vi "svfa_Compute Zoom FFT.vi"(0 "x":dbl[](array[numeric]) format="%.2f", 1 "processing control":T9(ring), 2 "spectrum info":T1={"channel name"="", "description"="", "x-axis units"=0, "spectral info"={"spectrum type"=enum."Power [Magnitude^2]", "linear/dB"=enum."linear", "window"=0, "window size"=0, "FFT size"=0}, "engineering units"=0, "custom label"="", "dB reference [EU]"=0.0, "peak units"=enum."rms", "weighting filter"=0, "spectral density?"=FALSE, "unit label"="", "spectrum skewed?"=FALSE, "complimentary spectrum units"=enum."none"} {"x-axis units" items=["Time (s)"=0, "Frequency-CB (Hz)"=1, "Frequency-CPB (Hz)"=1248, "Frequency-Arbitrary (Hz)"=2357, "Quefrency (s)"=2, "Revolutions (rev)"=3, "Order"=4, "Speed (RPM)"=11, "Speed (rad/s)"=21, "Index"=65535]; "weighting filter" items=["Linear", "A-weighting", "B-weighting", "C-weighting", "ITU-R 468-4", "Dolby", "CCITT", "C-message", "Wb", "Wc", "Wd", "We", "Wf", "Wh", "Wj", "Wk", "Wm", "AES17 20 kHz lowpass", "AES17 40 kHz lowpass", "AES17 20 kHz highpass", "AES17 40 kHz highpass"]; "dB reference [EU]" format="%.2f"; "engineering units" items=["custom..."=0, "V"=1, "A"=21, "C"=30, "pC"=31, "s"=32, "-"=29, "Pa"=2, "N"=20, "g"=3, "m/s^2"=4, "m/s"=5, "m"=6, "mm/s"=12, "mm"=13, "micron/s"=14, "micron"=15, "in/s^2"=7, "in/s"=8, "in"=9, "mil/s"=10, "mil"=11, "rad/s^2"=16, "rad/s"=17, "rad"=18, "deg/s^2"=26, "deg/s"=27, "deg"=28, "RPM"=22, "cycle/s^2"=23, "Hz"=24, "cycle"=25, "strain"=19]; "spectral info"."window" items=["None "=0, "Hanning"=1, "Hamming"=2, "Blackman-Harris"=3, "Exact Blackman"=4, "Blackman"=5, "Flat Top"=6, "4 Term B-Harris "=7, "7 Term B-Harris"=8, "Low Sidelobe"=9, "Force - Exponential"=10, "Gaussian"=62]}, 5 "fs":dbl=1024.0 format="%.2f", 9 "zoom FFT settings":T8={"zoom settings"={"center frequency"=-inf, "zoom"=1, "trim"=1.0}, "FFT settings"={"window"=enum."Hanning", "window size"=-1, "FFT size"=1024, "%overlap"=0.0}} {"FFT settings"."%overlap" min=0.0 max=100.0 format="%.2f"; "zoom settings"."trim" min=1.0 format="%.2f"; "zoom settings"."center frequency" format="%.2f"; "zoom settings"."zoom" min=1}, 11 "error in (no error)":errorcluster, 13 "export time data?":bool) -> (3 "spectrum info out":T1={"channel name"="", "description"="", "x-axis units"=0, "spectral info"={"spectrum type"=enum."Power [Magnitude^2]", "linear/dB"=enum."linear", "window"=0, "window size"=0, "FFT size"=0}, "engineering units"=0, "custom label"="", "dB reference [EU]"=0.0, "peak units"=enum."rms", "weighting filter"=0, "spectral density?"=FALSE, "unit label"="", "spectrum skewed?"=FALSE, "complimentary spectrum units"=enum."none"} {"x-axis units" items=["Time (s)"=0, "Frequency-CB (Hz)"=1, "Frequency-CPB (Hz)"=1248, "Frequency-Arbitrary (Hz)"=2357, "Quefrency (s)"=2, "Revolutions (rev)"=3, "Order"=4, "Speed (RPM)"=11, "Speed (rad/s)"=21, "Index"=65535]; "weighting filter" items=["Linear", "A-weighting", "B-weighting", "C-weighting", "ITU-R 468-4", "Dolby", "CCITT", "C-message", "Wb", "Wc", "Wd", "We", "Wf", "Wh", "Wj", "Wk", "Wm", "AES17 20 kHz lowpass", "AES17 40 kHz lowpass", "AES17 20 kHz highpass", "AES17 40 kHz highpass"]; "dB reference [EU]" format="%.2f"; "engineering units" items=["custom..."=0, "V"=1, "A"=21, "C"=30, "pC"=31, "s"=32, "-"=29, "Pa"=2, "N"=20, "g"=3, "m/s^2"=4, "m/s"=5, "m"=6, "mm/s"=12, "mm"=13, "micron/s"=14, "micron"=15, "in/s^2"=7, "in/s"=8, "in"=9, "mil/s"=10, "mil"=11, "rad/s^2"=16, "rad/s"=17, "rad"=18, "deg/s^2"=26, "deg/s"=27, "deg"=28, "RPM"=22, "cycle/s^2"=23, "Hz"=24, "cycle"=25, "strain"=19]; "spectral info"."window" items=["None "=0, "Hanning"=1, "Hamming"=2, "Blackman-Harris"=3, "Exact Blackman"=4, "Blackman"=5, "Flat Top"=6, "4 Term B-Harris "=7, "7 Term B-Harris"=8, "Low Sidelobe"=9, "Force - Exponential"=10, "Gaussian"=62]}, 4 "FFT spectrum":cluster{"f0":dbl, "df":dbl, "spectrum":cdb[]} {"spectrum" format="%.6g"; "df" format="%.2f"; "f0" format="%.2f"}, 10 "spectrum ready":bool, 14 "time data":T7 {"data" format="%.2f"; "dt" format="%.2f"; "t0" format="%.2f"}, 15 "error out":errorcluster)   [LabVIEW 2017]
doc: "This VI can only be in one case (zoom VIs cannot have a separate case for restart and for continue) within a caller. State maintained internally; first call primitives (ORed) with reset input reset filters, and the subVIs treat the first (filter length) samples as garbage."
uses:
  <vilib>/addons/_NISVFA/_Shared subVIs/Controls/svc_Spectrum Info.ctl
  <vilib>/addons/_NISVFA/_Shared subVIs/Controls/svc_X-Axis Units.ctl
  <vilib>/addons/_NISVFA/_Shared subVIs/Controls/svc_Spectrum Type.ctl
  <vilib>/addons/_NISVFA/_Shared subVIs/Controls/svc_Engineering Units Text Ring.ctl
  <vilib>/addons/_NISVFA/_Shared subVIs/Controls/svc_Weighting Filter Text Ring.ctl
  <vilib>/addons/_NISVFA/_Shared subVIs/Controls/svc_Complimentary Spectrum Units.ctl
  <vilib>/measure/masml.llb/ma_SML RT Baseband Zoom FFT (complex input).vi
  <vilib>/Analysis/sml.llb/aal_Complex Modulator(real input).vi
  <vilib>/Analysis/NI_AALPro.lvlib
  <vilib>/measure/NI_MAPro.lvlib
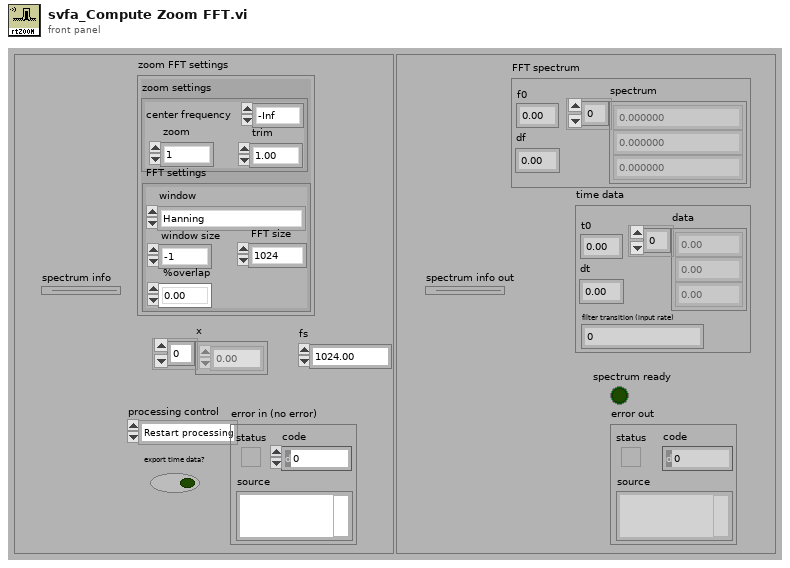
[diagram p1: front panel]
types:
  T1 = typedef "svc_Spectrum Info.ctl" = cluster{"channel name":string, "description":string, "x-axis units":T2, "spectral info":cluster{"spectrum type":T3, "linear/dB":enum16{"linear", "dB"}, "window":u16, "window size":i32, "FFT size":i32}, "engineering units":T4, "custom label":string, "dB reference [EU]":dbl, "peak units":enum16{"rms", "peak", "peak-peak"}, "weighting filter":T5, "spectral density?":bool, "unit label":string, "spectrum skewed?":bool, "complimentary spectrum units":T6}
  T2 = typedef "svc_X-Axis Units.ctl" = u16
  T3 = typedef "svc_Spectrum Type.ctl" = enum16{"FFT Spectrum [complex]", "Amplitude [Magnitude]", "Power [Magnitude^2]", "Cross Spectrum [complex]", "Frequency Response [Complex]"}
  T4 = typedef "svc_Engineering Units Text Ring.ctl" = u16
  T5 = typedef "svc_Weighting Filter Text Ring.ctl" = u16
  T6 = typedef "svc_Complimentary Spectrum Units.ctl" = enum16{"none", "radians", "degrees", "cycles", "imaginary"}
  T7 = cluster{"t0":dbl, "dt":dbl, "data":cdb[], "filter transition (input rate)":i32}
  T8 = cluster{"zoom settings":cluster{"center frequency":dbl, "zoom":i32, "trim":dbl}, "FFT settings":cluster{"window":enum16{"None ", "Hanning", "Hamming", "Blackman-Harris", "Exact Blackman", "Blackman", "Flat Top", "4 Term B-Harris ", "7 Term B-Harris", "Low Sidelobe"}, "window size":i32, "FFT size":i32, "%overlap":dbl}}
  T9 = enum16{"Restart processing", "Continue processing", "Skip processing"}
  T10 = cluster{"zoom":i32, "stop band attenuation":enum16{"84 dB", "96 dB", "120 dB"}, "alias protect in final transition":bool, "oversampling ratio":dbl}
  T11 = cluster{"x":dbl, "dt":dbl, "Time data":cdb[], "filter transition length":i32}
  T12 = cluster{"window":enum16{"None ", "Hanning", "Hamming", "Blackman-Harris", "Exact Blackman", "Blackman", "Flat Top", "4 Term B-Harris ", "7 Term B-Harris", "Low Sidelobe"}, "window size":i32, "FFT size":i32, "%overlap":dbl}
  T13 = typedef "NI_MAPro.lvlib/ma_sml_Spectral Info.ctl" = cluster{"spectrum type":enum16{"FFT Spectrum [complex]", "Amplitude [Magnitude]", "Power [Magnitude^2]", "Cross Spectrum [complex]", "Frequency Response [Complex]"}, "linear/dB":enum16{"linear", "dB"}, "window":u16, "window size":i32, "FFT size":i32}
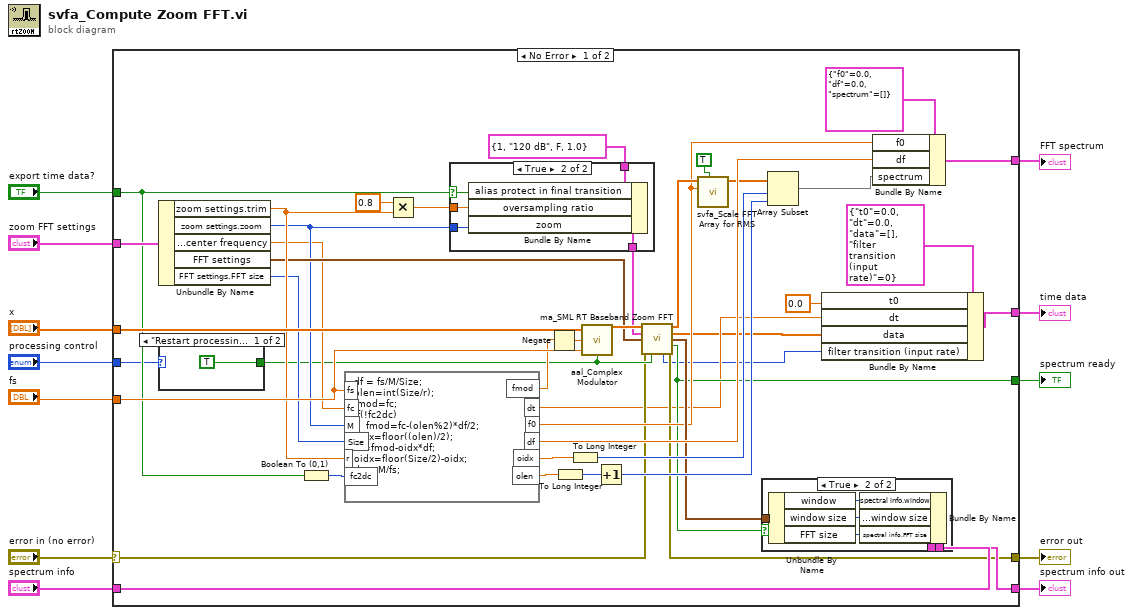
[diagram p0: block diagram]
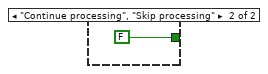
[diagram p3: hidden frame]
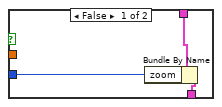
[diagram p4: hidden frame]
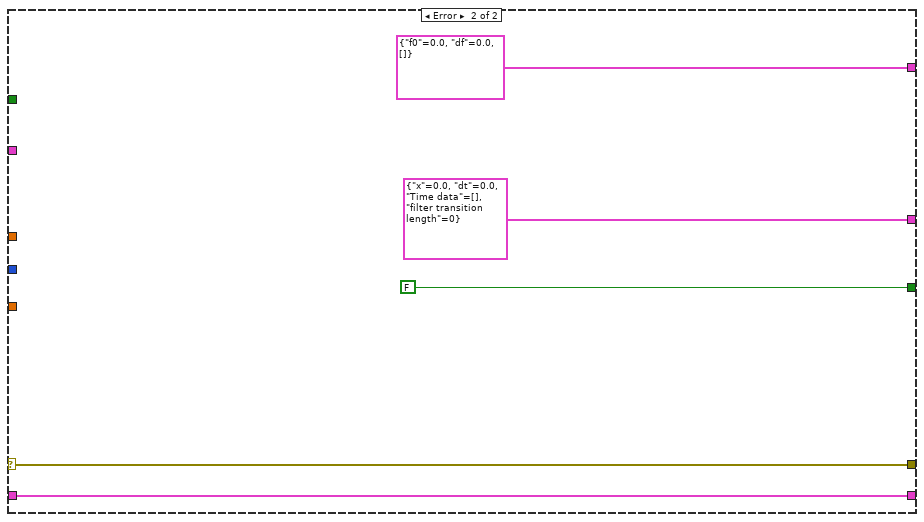
[diagram p5: hidden frame]
diagram:
  n1 = case shown="No Error" "error in (no error)" {
    selector: "error in (no error)" -> [w22 w75]
    tunnel: [w13 T11 {"x"=0.0, "dt"=0.0, "Time data"=[], "filter transition length"=0}] -> w7
    tunnel: [w20 FALSE ("SpectrumReady")] -> w12
    tunnel: "x" -> [w56 _]
    tunnel: "fs" -> [w54 _]
    tunnel: [w55 cluster{"f0":dbl, "df":dbl, cdb[]} {"f0"=0.0, "df"=0.0, []}] -> w10
    tunnel: "spectrum info" -> [w29 w74]
    tunnel: [w28 w74] -> w5
    tunnel: [w21 w75] -> w4
    tunnel: "zoom FFT settings" -> [w53 _]
    tunnel: "processing control" -> [w27 _]
    tunnel: "export time data?" -> [w52 _]
    frame No Error {
      n2 = Unbundle By Name(w53) -> ("zoom settings.trim"=w34:dbl, "zoom settings.zoom"=w31:i32, "zoom settings.center frequency"=w30:dbl, "FFT settings"=w32:T12, "FFT settings.FFT size"=w33:i32)
      n3 = case shown="\"Restart processing\", Default" w27 {
        tunnel: [TRUE FALSE] -> w23
        frame "Restart processing", Default {
        }
        frame "Continue processing", "Skip processing" {
        }
      }
      n4 = Boolean To (0,1)(Boolean=w52) -> (0, 1=w35:i16)
      n5 = formula code="df = fs/M/Size;\nolen=int(Size/r);\nfmod=fc;\nif(!fc2dc)\n    fmod=fc-(olen%2)*df/2;\noidx=floor((olen)/2);\nf0=fmod-oidx*df;\noidx=floor(Size/2)-oidx;\ndt = M/fs;"("fc"=w30, "M"=w31, "Size"=w33, "fs"=w54, "r"=w34, "fc2dc"=w35) -> ("f0"=w24:dbl, "df"=w49:dbl, "oidx"=w48:dbl, "olen"=w47:dbl, "dt"=w16:dbl, "fmod"=w36:dbl)
      n6 = Multiply(x=0.8, y=w34) -> (x*y=w40:dbl)
      n7 = case shown="True" w52 {
        selector: w52 -> [_ w71]
        tunnel: T10 {"zoom"=1, "stop band attenuation"=enum."120 dB", "alias protect in final transition"=FALSE, "oversampling ratio"=1.0} ("zoom settings") -> [w68 w73]
        tunnel: [w67 w72] -> w42
        tunnel: w31 -> [w66 w69]
        tunnel: w40 -> [_ w70]
        frame False {
          n8 = Bundle By Name(cluster=w68, "zoom"=w66) -> (w67:T10)
        }
        frame True {
          n9 = Bundle By Name(cluster=w73, "alias protect in final transition"=w71, "oversampling ratio"=w70, "zoom"=w69) -> (w72:T10)
        }
      }
      n10 = Negate(x=w36) -> (-x=w44:dbl)
      n11 = To Long Integer(number=w47) -> (32bit integer=w45:i32)
      n12 = To Long Integer(number=w48) -> (32bit integer=w46:i32)
      n13 = call-poly <vilib>:"aal_Complex Modulator.vi"("reset ?"=w23, "fs"=w54, "frequency"=w44, "x"=w56) -> ("y"=w50:cdb[])
      n14 = Increment(x=w45) -> (x+1=w41:i32)
      n15 = call-poly <vilib>:"ma_SML RT Baseband Zoom FFT.vi"("x [V]"=w50, "zoom settings"=w42, "FFT settings"=w32, "error in (no error)"=w22, "reset?"=w23) -> ("FFT{X} [Vrms]"=w51:cdb[], "time data"=w15:cdb[], "spectral info"=w26:T13, "spectrum ready?"=w20:bool, "filter transition length"=w14:i32, "error out"=w21:errorcluster)  [unwired: 5 in]
      n16 = call <vilib>:"svfa_Scale FFT Array for RMS.vi"("leave DC bin unscaled (T)"=TRUE, "f0"=w24, "FFT{X} [EU]"=w51) -> ("FFT {X} [rms]"=w38:cdb[])  [unwired: 8 in]
      n17 = case shown="True" w20 {
        tunnel: w29 -> [w57 w63]
        tunnel: [w57 w62] -> w28
        tunnel: w26 -> [_ w61]
        frame False {
        }
        frame True {
          n18 = Unbundle By Name(w61) -> ("window"=w60:u16, "window size"=w59:i32, "FFT size"=w58:i32)
          n19 = Bundle By Name(cluster=w63, "spectral info.window"=w60, "spectral info.window size"=w59, "spectral info.FFT size"=w58) -> (w62:T1)
        }
      }
      n20 = Array Subset(array=w38, index=w46, length=w41) -> (w37:cdb[])
      n21 = Bundle By Name(cluster=T7 {"t0"=0.0, "dt"=0.0, "data"=[], "filter transition (input rate)"=0} ("time data"), "t0"=0.0 ("x"), "dt"=w16, "data"=w15, "filter transition (input rate)"=w14) -> (w13:T7)
      n22 = Bundle By Name(cluster=cluster{"f0":dbl, "df":dbl, "spectrum":cdb[]} {"f0"=0.0, "df"=0.0, "spectrum"=[]} ("FFT spectrum"), "f0"=w24, "df"=w49, "spectrum"=w37) -> (w55:cluster{"f0":dbl, "df":dbl, "spectrum":cdb[]})
    }
    frame Error {
    }
  }
  "spectrum ready" <- w12
  "FFT spectrum" <- w10
  "error out" <- w4
  "time data" <- w7
  "spectrum info out" <- w5
